vi "giroscopio.vi"() -> ()   [LabVIEW 2016]
uses:
  <vilib>/MakerHub/LINX/Public/Sensors/Accelerometer/MPU60X0/GyroFullScaleRanges.ctl
  <vilib>/MakerHub/LINX/Public/Sensors/Accelerometer/MPU60X0/AccelFullScaleRanges.ctl
  <vilib>/MakerHub/LINX/Public/Sensors/Accelerometer/MPU60X0/Clock Source.ctl
  <vilib>/MakerHub/LINX/Public/Sensors/Accelerometer/MPU60X0/DeviceAddresses.ctl
  <vilib>/MakerHub/LINX/Public/Utilities/Open Serial.vi
  <vilib>/MakerHub/LINX/LMH-LINX.lvlib
  <vilib>/MakerHub/LINX/Public/Sensors/Accelerometer/MPU60X0/MPU60X0.lvlib
panel:
  out "Gyro  Data (dps)":T1
  out "Acceleration Data (g)":T1
  out "Giroscopio":T1(graph)
  out "Acelerometro":T1(graph)
  in  "Stop Button":bool
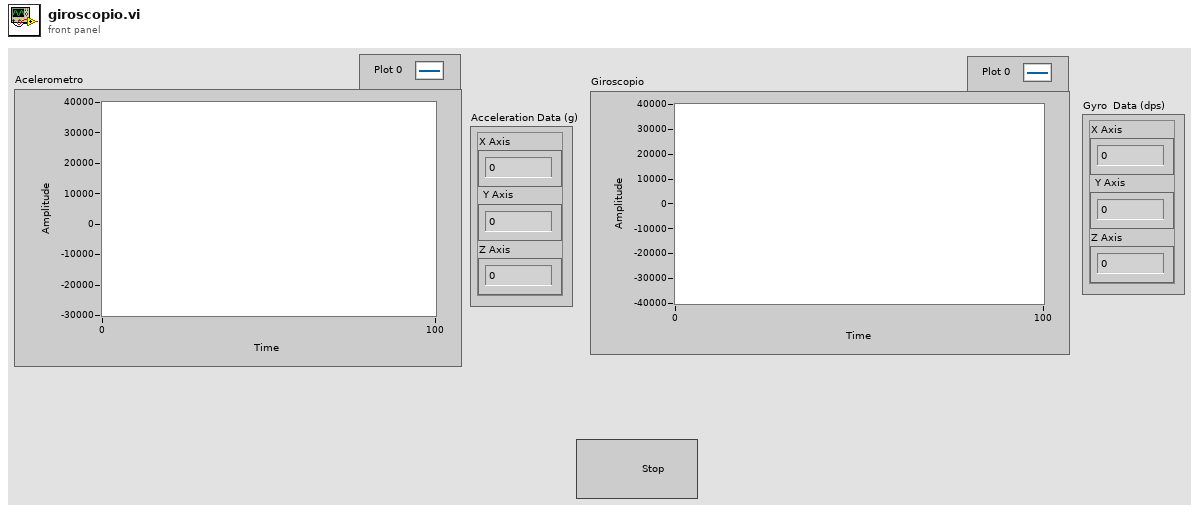
[diagram p1: front panel]
types:
  T1 = cluster{"X Axis":i16, "Y Axis":i16, "Z Axis":i16}
  T2 = typedef "LMH-LINX.lvlib/MPU60X0.lvlib/DeviceAddresses.ctl" = enum16{"0x68", "0x69"}
  T3 = typedef "LMH-LINX.lvlib/MPU60X0.lvlib/Clock Source.ctl" = enum8{"Internal 8MHz Osc", "PLL with X Gyro Ref", "PLL with Y Gyro Ref", "PLL with Z Gyro Ref", "PLL with ext 32.768 KHz Ref", "PLL with ext 19.2 MHz Ref", "Reserved", "Hold in reset"}
  T4 = typedef "LMH-LINX.lvlib/MPU60X0.lvlib/AccelFullScaleRanges.ctl" = enum16{"±2g", "±4g", "±8g", "±16g"}
  T5 = typedef "LMH-LINX.lvlib/MPU60X0.lvlib/GyroFullScaleRanges.ctl" = enum8{"±250 °/s", "±500 °/s", "±1000 °/s", "±2000 °/s"}
  T6 = typedef "LMH-LINX.lvlib/LINX Ref.ctl" = cluster{"IO":T7, "Interface":T8, "LINX Device Config":T9}
  T7 = typedef "LMH-LINX.lvlib/Platform.ctl" = enum16{"Remote", "Local"}
  T8 = typedef "LMH-LINX.lvlib/Interface.ctl" = enum16{"Serial", "TCP"}
  T9 = typedef "LMH-LINX.lvlib/Device.lvlib/LINX Device Config.ctl" = cluster{"Interface":T8, "COM Port":refnum<visa-resource-name>, "TCP Configuration":T10, "Device Family":u8, "Device ID":u8, "Device Name":string, "TCP Ref":refnum<k5>, "Channels":T11}
  T10 = typedef "LMH-LINX.lvlib/Device.lvlib/TCP Config.ctl" = cluster{"IP Address":string, "Port":u16}
  T11 = typedef "LMH-LINX.lvlib/Channels.ctl" = cluster{"DI":u8[], "DO":u8[], "AI":u8[], "AO":u8[], "PWM":u8[], "QE":u8[], "UART":u8[], "I2C 2":u8[], "SPI":u8[], "CAN":u8[], "Servo":u8[], "AI Ref (V)":dbl, "AI Resolution (Bits)":u8, "AO Ref (V)":dbl, "AO Resolution (Bits)":u8}
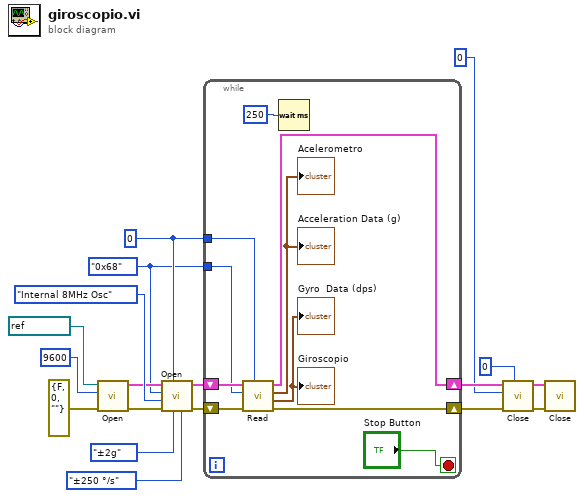
[diagram p0: block diagram]
diagram:
  w3 = DeviceAddresses."0x68" ("I2C Slave Address")
  w4 = u8 0 ("I2C Channel")
  n1 = call-poly <vilib>:"Open.vi"("Error In"=errorcluster {"status"=FALSE, "code"=0, "source"=""}, "Baud Rate Override"=u32 9600, "Serial Port"=refnum<visa-resource-name> "COM6") -> ("Error Out"=w7:errorcluster, "LINX Resource"=w8:T6)  [unwired: 6 in, 1 out]
  n2 = call <vilib>:"Open.vi"("Gyro Full Scale Range"=GyroFullScaleRanges."±250 °/s", "Accel Full Scale Range"=AccelFullScaleRanges."±2g", "I2C Channel"=w4, "Error In"=w7, "Clock Source"=Clock_Source."Internal 8MHz Osc", "I2C Slave Address"=w3, "LINX Resource"=w8) -> ("Error Out"=w5:errorcluster, "LINX Resource"=w6:T6)  [unwired: 3 in]
  n3 = while {
    tunnel: w3 -> [w20]
    tunnel: w4 -> [w19]
    shift-right: [w24] -> w12
    shift-left: w6 -> [w28]
    shift-right: [w23] -> w13
    shift-left: w5 -> [w21]
    stop <- "Stop Button" stop-if-true
    n4 = call <vilib>:"Read.vi"("I2C Channel"=w19, "Error In"=w21, "I2C Slave Address"=w20, "LINX Resource"=w28) -> ("Error Out"=w23:errorcluster, "Gyro  Data (dps)"=→"Giroscopio" →"Gyro  Data (dps)":T1, "Acceleration Data (g)"=→"Acelerometro" →"Acceleration Data (g)":T1, "LINX Resource"=w24:T6)  [unwired: 3 in, 1 out]
    n5 = Wait (ms)(milliseconds to wait=u32 250) -> ()  [unwired: 1 out]
  }
  n6 = call <vilib>:"Close.vi"("I2C Channel (0)"=u8 0, "Error In"=w13, "I2C Slave Address (0)"=u8 0, "LINX Resource"=w12) -> ("Error Out"=w15:errorcluster, "LINX Resource"=w14:T6)  [unwired: 6 in]
  n7 = call <vilib>:"Close.vi"("Error In"=w15, "LINX Resource"=w14) -> ()  [unwired: 9 in, 1 out]
